vi "create_user_event_stop.vi"(8 "error in (no error)":errorcluster caption="错误输入（无错误）") -> (0 "error out":errorcluster caption="错误输出", 2 "User Event - Stop":refnum<user-event> caption="用户事件－停止", 3 "Stop Event Registration Refnum":refnum<event-registration> caption="停止事件注册引用句柄")   [LabVIEW 2015, in "user_event_stop.lvlib"]
doc: "创建一个布尔用户事件，用于通过“消息处理循环”使“事件循环”停止执行。"
uses:
  user_event_stop.lvlib
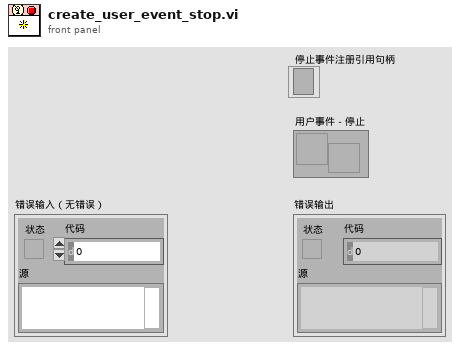
[diagram p1: front panel]
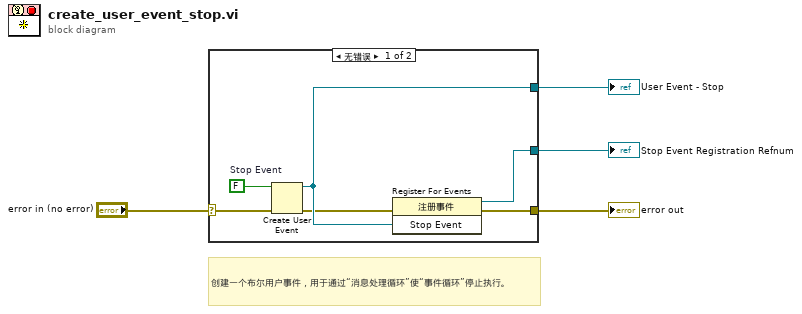
[diagram p0: block diagram]
diagram:
  # "创建一个布尔用户事件，用于通过“消息处理循环”使“事件循环”停止执行。"
  n1 = case shown="无错误" "error in (no error)" {
    selector: "error in (no error)" -> [w5 w11]
    tunnel: [w10 _] -> w4
    tunnel: [w9 _] -> w3
    tunnel: [w6 w11] -> w2
    frame No Error {
      w8 = FALSE  # Stop Event
      n2 = Create User Event(user event datatype=w8, error in=w5) -> (user event=w10:refnum<user-event>, error out=w7:errorcluster)
      n3 = register-events(error in=w7, w10) -> (reference out=w9:refnum<event-registration>, error out=w6:errorcluster)  [unwired: 1 in]
    }
    frame Error {
    }
  }
  "User Event - Stop" <- w4
  "error out" <- w2
  "Stop Event Registration Refnum" <- w3
